vi "Read Measurement Units.vi"(7 "Unit ID (A)":string="A", 8 "error in":errorcluster, 10 "Software Rev":u8, 11 "VISA Session In":refnum<visa-resource-name>="Alicat") -> (0 "error out":errorcluster, 1 "Lock Gas Select":bool, 2 "Measurement Units":T2, 3 "VISA Session Out":refnum<visa-resource-name>)   [LabVIEW 2023]
doc: "Reads the measurement units for the available variables. Measurement units are returned as strings."
panel:
  in  "Gauge (T) or \nDifferential (F)":bool
  out "Measurement Units Intermediate\n(newer revisions)":T1={"Abs. Pressure Units"=1, "Gauge/Diff. Press. Units"=1, "Barometric Press. Units"=1, "Temperature Units"=1, "Volumetric Units"=1, "Mass Units"=1, "Setpoint Units"=1, "Valve Drive Units"=1, "Total Mass Units"=1, "Total Volume Units"=1, "Time Units"=1} {"Setpoint Units" items=["Default"=0, "Unknown"=1, "SuL/m"=2, "SmL/s"=3, "SmL/m"=4, "SmL/h"=5, "SL/s"=6, "SLPM"=7, "SL/h"=8, "SCCS"=11, "SCCM"=12, "Scm3/h"=13, "Sm3/m"=14, "Sm3/h"=15, "Sm3/d"=16, "Sin3/m"=17, "SCFM"=18, "SCFH"=19, "kSCFM"=20, "NuL/m"=32, "NmL/s"=33, "NmL/m"=34, "NmL/h"=35, "NL/s"=36, "NLPM"=37, "NL/h"=38, "NCCS"=41, "NCCM"=42, "Ncm3/h"=43, "Nm3/m"=44, "Nm3/h"=45, "Nm3/d"=46, "count"=62, "%"=63, "mg/s"=64, "mg/m"=65, "g/s"=66, "g/m"=67, "g/h"=68, "kg/m"=69, "kg/h"=70, "oz/s"=71, "oz/m"=72, "lb/m"=73, "lb/h"=74]; "Barometric Press. Units" items=["Default"=0, "Unknown"=1, "Pa"=2, "hPa"=3, "kPa"=4, "MPa"=5, "mbar"=6, "bar"=7, "g/cm2"=8, "kg/cm"=9, "PSI"=10, "PSF"=11, "mTorr"=12, "torr"=13, "mmHg"=14, "inHg"=15, "mmH2O"=16, "mmH2O"=17, "cmH2O"=18, "cmH2O"=19, "inH2O"=20, "inH2O"=21, "atm"=22, "m asl"=23, "ft asl"=24, "V"=61, "count"=62, "%"=63]; "Gauge/Diff. Press. Units" items=["Default"=0, "Unknown"=1, "Pa"=2, "hPa"=3, "kPa"=4, "MPa"=5, "mbar"=6, "bar"=7, "g/cm2"=8, "kg/cm"=9, "PSI"=10, "PSF"=11, "mTorr"=12, "torr"=13, "mmHg"=14, "inHg"=15, "mmH2O"=16, "mmH2O"=17, "cmH2O"=18, "cmH2O"=19, "inH2O"=20, "inH2O"=21, "atm"=22, "m asl"=23, "ft asl"=24, "V"=61, "count"=62, "%"=63]; "Time Units" items=["Default", "Unknown", "h:m:s", "ms", "s", "m", "hour", "day"]; "Total Volume Units" items=["Default"=0, "Unknown"=1, "uL"=2, "mL"=3, "L"=4, "US GAL"=5, "cm3"=6, "m3"=7, "in3"=8, "ft3"=9, "uP"=61]; "Total Mass Units" items=["Default"=0, "Unknown"=1, "SuL"=2, "SmL"=3, "SL"=4, "Scm3"=6, "Sm3"=7, "Sin3"=8, "Sft3"=9, "kSft3"=10, "NuL"=32, "NmL"=33, "NL"=34, "Ncm3"=35, "Nm3"=36, "mg"=64, "g"=65, "kg"=66, "oz"=67, "lb"=68]; "Valve Drive Units" items=["Default"=0, "Unknown"=1, "count"=2, "%"=63]; "Mass Units" items=["Default"=0, "Unknown"=1, "SuL/m"=2, "SmL/s"=3, "SmL/m"=4, "SmL/h"=5, "SL/s"=6, "SLPM"=7, "SL/h"=8, "SCCS"=11, "SCCM"=12, "Scm3/h"=13, "Sm3/m"=14, "Sm3/h"=15, "Sm3/d"=16, "Sin3/m"=17, "SCFM"=18, "SCFH"=19, "kSCFM"=20, "NuL/m"=32, "NmL/s"=33, "NmL/m"=34, "NmL/h"=35, "NL/s"=36, "NLPM"=37, "NL/h"=38, "NCCS"=41, "NCCM"=42, "Ncm3/h"=43, "Nm3/m"=44, "Nm3/h"=45, "Nm3/d"=46, "count"=62, "%"=63, "mg/s"=64, "mg/m"=65, "g/s"=66, "g/m"=67, "g/h"=68, "kg/m"=69, "kg/h"=70, "oz/s"=71, "oz/m"=72, "lb/m"=73, "lb/h"=74]; "Volumetric Units" items=["Default"=0, "Unknown"=1, "uL/m"=2, "mL/s"=3, "mL/m"=4, "mL/h"=5, "L/s"=6, "LPM"=7, "L/h"=8, "US GPM"=9, "US GPH"=10, "CCS"=11, "CCM"=12, "cm3/h"=13, "m3/m"=14, "m3/h"=15, "m3/d"=16, "in3/m"=17, "CFM"=18, "CFH"=19, "count"=62, "%"=63]; "Temperature Units" items=["Default", "Unknown", "°C", "°F", "K", "°Ra"]; "Abs. Pressure Units" items=["Default"=0, "Unknown"=1, "Pa"=2, "hPa"=3, "kPa"=4, "MPa"=5, "mbar"=6, "bar"=7, "g/cm2"=8, "kg/cm"=9, "PSI"=10, "PSF"=11, "mTorr"=12, "torr"=13, "mmHg"=14, "inHg"=15, "mmH2O"=16, "mmH2O"=17, "cmH2O"=18, "cmH2O"=19, "inH2O"=20, "inH2O"=21, "atm"=22, "m asl"=23, "ft asl"=24, "V"=61, "count"=62, "%"=63]}
  out "Measurement Units Intermediate\n(older revisions)":T3={"Pressure Units"=0, "Mass Units"=0, "Temperature Units"=0, "Volume Units"=0, "Totalizer Units"=15, "Totalizer Avg Units"=15} {"Totalizer Units" items=["CC", "uL", "L", "CI", "CF", "CM", "GAL", "mL", "uP", "Lbs", "N/A", "N/A", "N/A", "SCC", "SuL", "SL", "SCI", "SCF", "NCM", "Grams", "Kg", "Lbs", "mg", "SCM", "SmL", "KSCF"]; "Totalizer Avg Units" items=["CCM", "uLPM", "LPM", "CIM", "CFM", "CM/M", "GAL/M", "mLPM", "uP/M", "Lbs/M", "N/A", "N/A", "N/A", "SCCM", "SuLPM", "SLPM", "SCIM", "SCFM", "NCM/M", "Grams/M", "Kg/M", "Lbs/M", "mg/M", "SCM/M", "SmLPM", "KSCFM"]; "Volume Units" items=["CCM"=0, "CCH"=64, "uLPM"=256, "LPS"=320, "LPM"=512, "CM/D"=576, "CIM"=768, "Percent"=832, "CFH"=1024, "Kg/M"=1088, "CM/H"=1280, "Kg/H"=1344, "CFM"=1536, "mLPS"=1600, "GPM"=1792, "CCS"=1856, "GPH"=2048, "mLPH"=2112, "Grams/S"=2304, "Lbs/H"=2368, "Grams/M"=2560, "Grams/H"=2816, "mg/M"=3072, "LPH"=3328, "oz/S"=3584, "mLPM"=3840]; "Temperature Units" items=["C"=0, "K"=16, "F"=32, "R"=48]; "Mass Units" items=["SCCM"=0, "SLPH"=128, "SuLPM"=4096, "SmLPM"=4224, "SLPM"=8192, "Grams/S"=8320, "SCIM"=12288, "SCM/H"=12416, "SCFH"=16384, "SCCH"=16512, "NCM/H"=20480, "NLPH"=20608, "SCFM"=24576, "NLPS"=24704, "Grams/M"=28672, "SCM/D"=28800, "Grams/H"=32768, "NmLPM"=32896, "Kg/M"=36864, "SCCS"=36992, "Kg/H"=40960, "NmLPH"=41088, "Lbs/M"=45056, "SLPS"=45184, "Lbs/H"=49152, "SmLPS"=49280, "mg/M"=53248, "mg/S"=53376, "NLPM"=57344, "NCCM"=61440]; "Pressure Units" items=["PSI", "PSI", "Torr", "Bar", "mBar", "Pascal", "KPa", "MPa", "inHg", "mmHg", "inH2O", "PSID", "mTorr", "cmH2O", "Kg/CM2", "mmH2O"]}
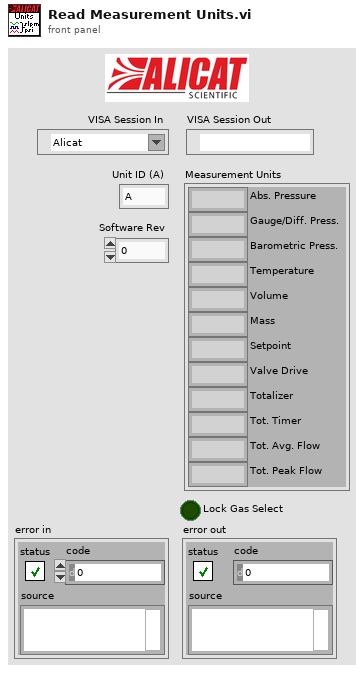
[diagram p1: front panel]
types:
  T1 = cluster{"Abs. Pressure Units":u16, "Gauge/Diff. Press. Units":u16, "Barometric Press. Units":u16, "Temperature Units":u16, "Volumetric Units":u16, "Mass Units":u16, "Setpoint Units":u16, "Valve Drive Units":u16, "Total Mass Units":u16, "Total Volume Units":u16, "Time Units":u16}
  T2 = cluster{"Abs. Pressure":string, "Gauge/Diff. Press.":string, "Barometric Press.":string, "Temperature":string, "Volume":string, "Mass":string, "Setpoint":string, "Valve Drive":string, "Totalizer":string, "Tot. Timer":string, "Tot. Avg. Flow":string, "Tot. Peak Flow":string}
  T3 = cluster{"Pressure Units":i32, "Mass Units":i32, "Temperature Units":i32, "Volume Units":i32, "Totalizer Units":u16, "Totalizer Avg Units":u16}
  T4 = cluster{"Pressure":i32, "Mass":i32, "Temperature":i32, "Volume":i32, "Totalizer Units":u16, "Totalizer Avg Units":u16}
  T5 = typedef "LVStringsAndValuesArrayTypeDef_U16.ctl" = cluster{"String":string, "Value":u16}[]
  T6 = cluster{"Controller Select":u16, "SetPoint Source":enum8{"Serial", "Local", "Analog", "Unknown"}, "AutoTare":enum16{"Disabled", "Enabled"}}
  T7 = typedef "LVStringsAndValuesArrayTypeDef_I32.ctl" = cluster{"String":string, "Value":i32}[]
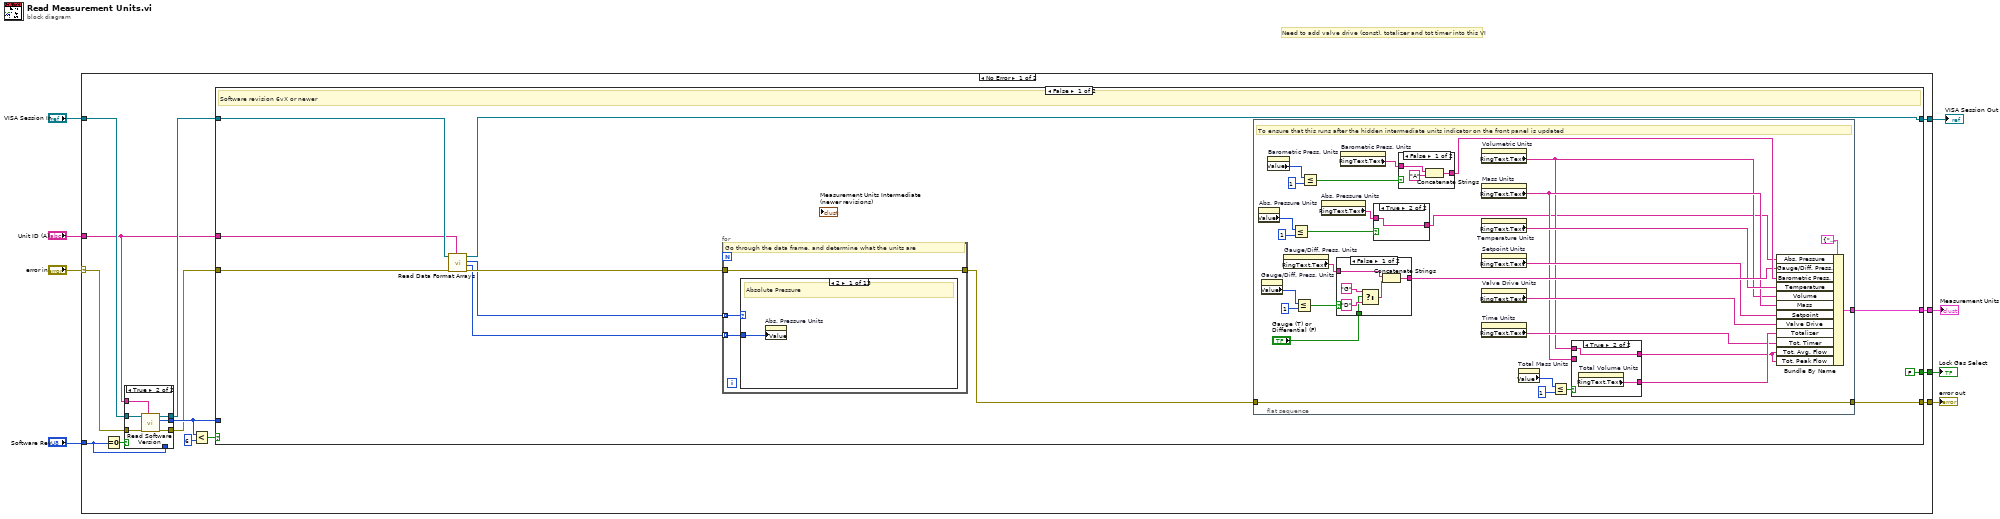
[diagram p0: block diagram]
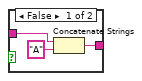
[diagram p5: hidden frame]
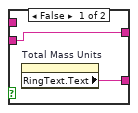
[diagram p6: hidden frame]
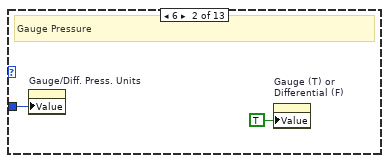
[diagram p7: hidden frame]
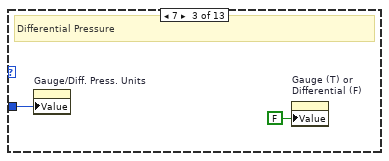
[diagram p8: hidden frame]
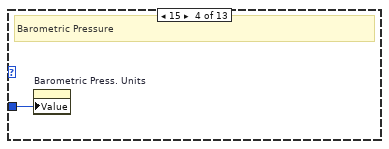
[diagram p9: hidden frame]
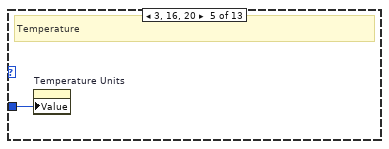
[diagram p10: hidden frame]
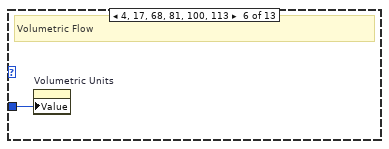
[diagram p11: hidden frame]
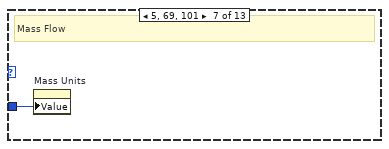
[diagram p12: hidden frame]
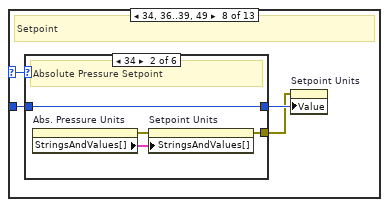
[diagram p13: hidden frame]
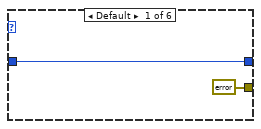
[diagram p14: hidden frame]
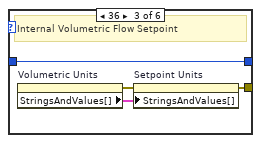
[diagram p15: hidden frame]
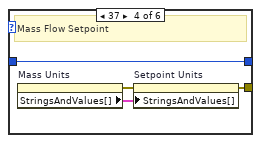
[diagram p16: hidden frame]
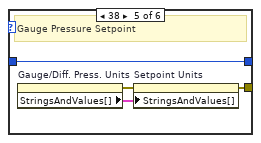
[diagram p17: hidden frame]
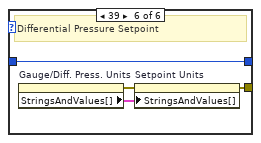
[diagram p18: hidden frame]
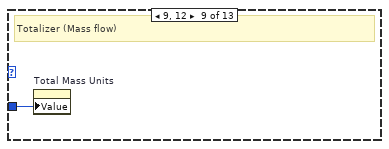
[diagram p19: hidden frame]
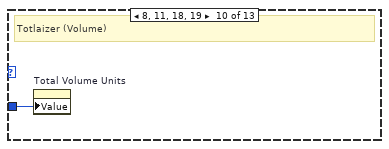
[diagram p20: hidden frame]
diagram:
  # "Need to add valve drive (const), totalizer and tot timer into this VI"
  n1 = case shown="No Error" "error in" {
    selector: "error in" -> [w11 w253]
    tunnel: [w22 TRUE ("Lock Gas Select")] -> w8
    tunnel: [w21 w253] -> w7
    tunnel: "Software Rev" -> [w15 _]
    tunnel: "Unit ID (A)" -> [w9 _]
    tunnel: "VISA Session In" -> [w10 w256]
    tunnel: [w19 w256] -> w3
    tunnel: [w18 T2 {"Abs. Pressure"="", "Gauge/Diff. Press."="", "Barometric Press."="", "Temperature"="", "Volume"="", "Mass"="", "Setpoint"="", "Valve Drive"="", "Totalizer"="", "Tot. Timer"="", "Tot. Avg. Flow"="", "Tot. Peak Flow"=""} ("Measurement Units")] -> w2
    frame No Error {
      n2 = Equal To 0?(x=w15) -> (x = 0?=w16:bool)
      n3 = case shown="True" w16 {
        tunnel: w11 -> [w24 w31]
        tunnel: w10 -> [w23 w30]
        tunnel: w9 -> [_ w29]
        tunnel: [w24 w28] -> w12
        tunnel: [w23 w27] -> w13
        tunnel: [w25 w26] -> w14
        tunnel: w15 -> [w25 _]
        frame False {
        }
        frame True {
          n4 = call "Read Software Version.vi"("Unit ID (A)"=w29, "error in"=w31, "VISA Session In"=w30) -> ("error out"=w28:errorcluster, "Software Version"=w26:u8, "VISA Session Out"=w27:refnum<visa-resource-name>)  [unwired: 6 in]
        }
      }
      n5 = Less?(x=w14, y=u8 6) -> (x < y?=w20:bool)
      n6 = case shown="False" w20 {
        tunnel: [FALSE ("Lock Gas Select") w157] -> w22
        tunnel: w12 -> [w38 w148]
        tunnel: [w40 w143] -> w21
        tunnel: w14 -> [_ w152]
        tunnel: w13 -> [w37 w149]
        tunnel: w9 -> [w36 w138]
        tunnel: [w35 w145] -> w19
        tunnel: [w39 w144] -> w18
        frame False {
          # "Software revision 6vX or newer"
          n7 = call "Read Data Format Arrays.vi"("Unit ID (A)"=w36, "error in (no error)"=w38, "VISA Session In"=w37) -> ("error out"=w34:errorcluster, "Units Array"=w32:u16[], "Data Type Array"=w33:u16[], "VISA Session Out"=w35:refnum<visa-resource-name>)  [unwired: 5 in]
          n8 = for {
            tunnel: w32 -> [w93] mode=indexing
            tunnel: w33 -> [w94] mode=indexing
            tunnel: [w92] -> w41
            tunnel: w34 -> [w92]
            # "Go through the data frame, and determine what the units are"
            n9 = case shown="2" w94 {
              selector: w94 -> [_ _ _ _ _ _ _ w105 _ _ _ _ _]
              tunnel: w93 -> [w95 w97 w99 w100 w101 w102 w103 w104 w130 w131 w132 w133 _]
              frame 2 {
                # "Absolute Pressure"
                n10 = property on="Abs. Pressure Units" class="Ring (strict)"("Value"=w95) -> ()  [unwired: 2 in, 2 out]
              }
              frame 6 {
                # "Gauge Pressure"
                n11 = property on="Gauge/Diff. Press. Units" class="Ring (strict)"("Value"=w97) -> ()  [unwired: 2 in, 2 out]
                n12 = property on="Gauge (T) or \nDifferential (F)" class="Bool (strict)"("Value"=TRUE ("Gauge")) -> ()  [unwired: 2 in, 2 out]
              }
              frame 7 {
                # "Differential Pressure"
                n13 = property on="Gauge/Diff. Press. Units" class="Ring (strict)"("Value"=w99) -> ()  [unwired: 2 in, 2 out]
                n14 = property on="Gauge (T) or \nDifferential (F)" class="Bool (strict)"("Value"=FALSE ("Gauge")) -> ()  [unwired: 2 in, 2 out]
              }
              frame 15 {
                # "Barometric Pressure"
                n15 = property on="Barometric Press. Units" class="Ring (strict)"("Value"=w100) -> ()  [unwired: 2 in, 2 out]
              }
              frame 3, 16, 20 {
                # "Temperature"
                n16 = property on="Temperature Units" class="Ring (strict)"("Value"=w101) -> ()  [unwired: 2 in, 2 out]
              }
              frame 4, 17, 68, 81, 100, 113 {
                # "Volumetric Flow"
                n17 = property on="Volumetric Units" class="Ring (strict)"("Value"=w102) -> ()  [unwired: 2 in, 2 out]
              }
              frame 5, 69, 101 {
                # "Mass Flow"
                n18 = property on="Mass Units" class="Ring (strict)"("Value"=w103) -> ()  [unwired: 2 in, 2 out]
              }
              frame 34, 36..39, 49 {
                # "Setpoint"
                n19 = case shown="34" w105 {
                  tunnel: [w108 w110 w114 w118 w122 w126] -> w107
                  tunnel: [errorcluster {"status"=FALSE, "code"=0, "source"=""} ("error out") w111 w115 w119 w123 w127] -> w106
                  tunnel: w104 -> [w108 w110 w114 w118 w122 w126]
                  frame Default {
                  }
                  frame 34 {
                    # "Absolute Pressure Setpoint"
                    n20 = property on="Abs. Pressure Units" class="Ring (strict)"() -> (error out=w113:errorcluster, "StringsAndValues[]"=w112:T5)  [unwired: 2 in, 1 out]
                    n21 = property on="Setpoint Units" class="Ring (strict)"(error in=w113, "StringsAndValues[]"=w112) -> (error out=w111:errorcluster)  [unwired: 1 in, 1 out]
                  }
                  frame 36 {
                    # "Internal Volumetric Flow Setpoint"
                    n22 = property on="Volumetric Units" class="Ring (strict)"() -> (error out=w117:errorcluster, "StringsAndValues[]"=w116:T5)  [unwired: 2 in, 1 out]
                    n23 = property on="Setpoint Units" class="Ring (strict)"(error in=w117, "StringsAndValues[]"=w116) -> (error out=w115:errorcluster)  [unwired: 1 in, 1 out]
                  }
                  frame 37 {
                    # "Mass Flow Setpoint"
                    n24 = property on="Mass Units" class="Ring (strict)"() -> (error out=w121:errorcluster, "StringsAndValues[]"=w120:T5)  [unwired: 2 in, 1 out]
                    n25 = property on="Setpoint Units" class="Ring (strict)"(error in=w121, "StringsAndValues[]"=w120) -> (error out=w119:errorcluster)  [unwired: 1 in, 1 out]
                  }
                  frame 38 {
                    # "Gauge Pressure Setpoint"
                    n26 = property on="Gauge/Diff. Press. Units" class="Ring (strict)"() -> (error out=w125:errorcluster, "StringsAndValues[]"=w124:T5)  [unwired: 2 in, 1 out]
                    n27 = property on="Setpoint Units" class="Ring (strict)"(error in=w125, "StringsAndValues[]"=w124) -> (error out=w123:errorcluster)  [unwired: 1 in, 1 out]
                  }
                  frame 39 {
                    # "Differential Pressure Setpoint"
                    n28 = property on="Gauge/Diff. Press. Units" class="Ring (strict)"() -> (error out=w129:errorcluster, "StringsAndValues[]"=w128:T5)  [unwired: 2 in, 1 out]
                    n29 = property on="Setpoint Units" class="Ring (strict)"(error in=w129, "StringsAndValues[]"=w128) -> (error out=w127:errorcluster)  [unwired: 1 in, 1 out]
                  }
                }
                n30 = property on="Setpoint Units" class="Ring (strict)"(error in=w106, "Value"=w107) -> ()  [unwired: 1 in, 2 out]
              }
              frame 9, 12 {
                # "Totalizer (Mass flow)"
                n31 = property on="Total Mass Units" class="Ring (strict)"("Value"=w130) -> ()  [unwired: 2 in, 2 out]
              }
              frame 8, 11, 18, 19 {
                # "Totlaizer (Volume)"
                n32 = property on="Total Volume Units" class="Ring (strict)"("Value"=w131) -> ()  [unwired: 2 in, 2 out]
              }
              frame 13 {
                # "Valve Drive"
                n33 = property on="Valve Drive Units" class="Ring (strict)"("Value"=w132) -> ()  [unwired: 2 in, 2 out]
              }
              frame 10, 14 {
                # "Time"
                n34 = property on="Time Units" class="Ring (strict)"("Value"=w133) -> ()  [unwired: 2 in, 2 out]
              }
              frame Default {
              }
            }
          }
          n35 = flat-sequence {
            tunnel: w41 -> [w59]
            tunnel: [w59] -> w40
            tunnel: [w44] -> w39
            frame #0 {
              # "To ensure that this runs after the hidden intermediate units indicator on the front panel is updated"
              n36 = property on="Abs. Pressure Units" class="Ring (strict)"() -> ("Value"=w65:u16)  [unwired: 2 in, 2 out]
              n37 = property on="Gauge/Diff. Press. Units" class="Ring (strict)"() -> ("Value"=w66:u16)  [unwired: 2 in, 2 out]
              n38 = property on="Barometric Press. Units" class="Ring (strict)"() -> ("Value"=w69:u16)  [unwired: 2 in, 2 out]
              n39 = property on="Gauge/Diff. Press. Units" class="Ring (strict)"() -> ("RingText.Text"=w56:string)  [unwired: 2 in, 2 out]
              n40 = Less Or Equal?(x=w65, y=u16 1) -> (x <= y?=w63:bool)
              n41 = Less Or Equal?(x=w66, y=u16 1) -> (x <= y?=w57:bool)
              n42 = Less Or Equal?(x=w69, y=u16 1) -> (x <= y?=w60:bool)
              n43 = property on="Abs. Pressure Units" class="Ring (strict)"() -> ("RingText.Text"=w62:string)  [unwired: 2 in, 2 out]
              n44 = case shown="False" w57 {
                tunnel: w56 -> [w78 w79]
                tunnel: [w77 w79] -> w54
                tunnel: "Gauge (T) or \nDifferential (F)" -> [w73 _]
                frame False {
                  n45 = Select(t="G" ("string"), s=w73, f="D" ("string")) -> (s? t:f=w74:string)
                  n46 = Concatenate Strings(w78, w74) -> (w77:string)
                }
                frame True {
                }
              }
              n47 = property on="Barometric Press. Units" class="Ring (strict)"() -> ("RingText.Text"=w61:string)  [unwired: 2 in, 2 out]
              n48 = case shown="True" w63 {
                tunnel: w62 -> [w85 w87]
                tunnel: [w84 w87] -> w43
                frame False {
                  n49 = Concatenate Strings(w85, "A" ("string")) -> (w84:string)
                }
                frame True {
                }
              }
              n50 = case shown="False" w60 {
                tunnel: w61 -> [w81 w83]
                tunnel: [w80 w83] -> w55
                frame False {
                  n51 = Concatenate Strings(w81, "A" ("string")) -> (w80:string)
                }
                frame True {
                }
              }
              n52 = property on="Volumetric Units" class="Ring (strict)"() -> ("RingText.Text"=w46:string)  [unwired: 2 in, 2 out]
              n53 = property on="Mass Units" class="Ring (strict)"() -> ("RingText.Text"=w47:string)  [unwired: 2 in, 2 out]
              n54 = property on="Temperature Units" class="Ring (strict)"() -> ("RingText.Text"=w53:string)  [unwired: 2 in, 2 out]
              n55 = property on="Setpoint Units" class="Ring (strict)"() -> ("RingText.Text"=w50:string)  [unwired: 2 in, 2 out]
              n56 = property on="Valve Drive Units" class="Ring (strict)"() -> ("RingText.Text"=w49:string)  [unwired: 2 in, 2 out]
              n57 = property on="Time Units" class="Ring (strict)"() -> ("RingText.Text"=w48:string)  [unwired: 2 in, 2 out]
              n58 = property on="Total Mass Units" class="Ring (strict)"() -> ("Value"=w70:u16)  [unwired: 2 in, 2 out]
              n59 = Less Or Equal?(x=w70, y=u16 1) -> (x <= y?=w71:bool)
              n60 = case shown="True" w71 {
                tunnel: [w89 w91] -> w51
                tunnel: w47 -> [w88 _]
                tunnel: w46 -> [_ w90]
                tunnel: [w88 w90] -> w45
                frame False {
                  n61 = property on="Total Mass Units" class="Ring (strict)"() -> ("RingText.Text"=w89:string)  [unwired: 2 in, 2 out]
                }
                frame True {
                  n62 = property on="Total Volume Units" class="Ring (strict)"() -> ("RingText.Text"=w91:string)  [unwired: 2 in, 2 out]
                }
              }
              n63 = Bundle By Name(cluster=T2 {"Abs. Pressure"="", "Gauge/Diff. Press."="", "Barometric Press."="", "Temperature"="", "Volume"="", "Mass"="", "Setpoint"="", "Valve Drive"="", "Totalizer"="", "Tot. Timer"="", "Tot. Avg. Flow"="", "Tot. Peak Flow"=""} ("Measurement Units"), "Abs. Pressure"=w43, "Gauge/Diff. Press."=w54, "Barometric Press."=w55, "Temperature"=w53, "Volume"=w46, "Mass"=w47, "Setpoint"=w50, "Valve Drive"=w49, "Totalizer"=w51, "Tot. Timer"=w48, "Tot. Avg. Flow"=w45, "Tot. Peak Flow"=w45) -> (w44:T2)
            }
          }
        }
        frame True {
          # "If true mass units on an \nold board: lock gas select"
          # "Software revision 5vX or older"
          n64 = call "Read Register.vi"("Unit ID (A)"=w138, "error in"=w148, "Register address"=u16 45, "VISA Session In"=w149) -> ("error out"=w142:errorcluster, "Register Value (I32)"=w147:i32, "VISA Session Out"=w140:refnum<visa-resource-name>)  [unwired: 5 in]
          n65 = call "Read Output Definitions and Controller Options.vi"("Unit ID (A)"=w138, "error in"=w142, "VISA Session In"=w140) -> ("error out"=w141:errorcluster, "Read/Write Options"=w137:T6, "VISA Session Out"=w139:refnum<visa-resource-name>)  [unwired: 5 in, 1 out]
          n66 = Unbundle By Name(w137) -> ("Controller Select"=w136:u16)
          n67 = call "Read Totalizer Units and Decimals.vi"("Unit ID (A)"=w138, "error in"=w141, "VISA Session In"=w139) -> ("error out"=w146:errorcluster, "Totalizer Units"=w135:string, "VISA Session Out"=w145:refnum<visa-resource-name>)  [unwired: 4 in, 2 out]
          n68 = property on="Mass Units" class="Ring (strict)"(error in=w146) -> (error out=w156:errorcluster, "StringsAndValues[]"=w194:T7)  [unwired: 1 in, 1 out]
          n69 = for {
            tunnel: w194 -> [w252] mode=indexing
            tunnel: [w251] -> w170 mode=indexing
            n70 = Unbundle By Name(w252) -> ("Value"=w251:i32)
          }
          n71 = property on="Volume Units" class="Ring (strict)"(error in=w156) -> (error out=w155:errorcluster, "StringsAndValues[]"=w185:T7)  [unwired: 1 in, 1 out]
          n72 = Less Or Equal?(x=w170, y=w147) -> (x <= y?=w193:bool[])
          n73 = Boolean To (0,1)(Boolean=w193) -> (0, 1=w192:i16[])
          n74 = To Long Integer(number=w192) -> (32bit integer=w191:i32[])
          n75 = Multiply(x=w170, y=w191) -> (x*y=w190:i32[])
          n76 = for {
            tunnel: w185 -> [w250] mode=indexing
            tunnel: [w249] -> w168 mode=indexing
            n77 = Unbundle By Name(w250) -> ("Value"=w249:i32)
          }
          n78 = Array Max & Min(array=w190) -> (max value=w164:i32, max index (indices)=w169:i32)  [unwired: 2 out]
          n79 = Subtract(x=w147, y=w164) -> (x-y=w184:i32)
          n80 = property on="Temperature Units" class="Ring (strict)"(error in=w155) -> (error out=w154:errorcluster, "StringsAndValues[]"=w183:T7)  [unwired: 1 in, 1 out]
          n81 = Less Or Equal?(x=w168, y=w184) -> (x <= y?=w186:bool[])
          n82 = Boolean To (0,1)(Boolean=w186) -> (0, 1=w187:i16[])
          n83 = To Long Integer(number=w187) -> (32bit integer=w188:i32[])
          n84 = Multiply(x=w168, y=w188) -> (x*y=w189:i32[])
          n85 = for {
            tunnel: w183 -> [w248] mode=indexing
            tunnel: [w247] -> w167 mode=indexing
            n86 = Unbundle By Name(w248) -> ("Value"=w247:i32)
          }
          n87 = Array Max & Min(array=w189) -> (max value=w163:i32)  [unwired: 3 out]
          n88 = Subtract(x=w184, y=w163) -> (x-y=w173:i32)
          n89 = property on="Pressure Units" class="Ring (strict)"(error in=w154) -> (error out=w153:errorcluster, "StringsAndValues[]"=w174:T7)  [unwired: 1 in, 1 out]
          n90 = Less Or Equal?(x=w167, y=w173) -> (x <= y?=w182:bool[])
          n91 = Boolean To (0,1)(Boolean=w182) -> (0, 1=w181:i16[])
          n92 = To Long Integer(number=w181) -> (32bit integer=w180:i32[])
          n93 = Multiply(x=w167, y=w180) -> (x*y=w179:i32[])
          n94 = for {
            tunnel: w174 -> [w246] mode=indexing
            tunnel: [w245] -> w166 mode=indexing
            n95 = Unbundle By Name(w246) -> ("Value"=w245:i32)
          }
          n96 = Array Max & Min(array=w179) -> (max value=w162:i32)  [unwired: 3 out]
          n97 = Subtract(x=w173, y=w162) -> (x-y=w172:i32)
          n98 = Less Or Equal?(x=w166, y=w172) -> (x <= y?=w175:bool[])
          n99 = Boolean To (0,1)(Boolean=w175) -> (0, 1=w176:i16[])
          n100 = To Long Integer(number=w176) -> (32bit integer=w177:i32[])
          n101 = Multiply(x=w166, y=w177) -> (x*y=w178:i32[])
          n102 = Array Max & Min(array=w178) -> (max value=w161:i32)  [unwired: 3 out]
          n103 = Subtract(x=w172, y=w161) -> (x-y=w171:i32)
          n104 = Not Equal To 0?(x=w171) -> (x != 0?=w165:bool)
          n105 = case shown="True" w165 {
            tunnel: w170 -> [_ w244]
            tunnel: w169 -> [_ w242]
            tunnel: w168 -> [_ w237]
            tunnel: w167 -> [_ w231]
            tunnel: w166 -> [_ w225]
            tunnel: w164 -> [w218 _]
            tunnel: w163 -> [w217 _]
            tunnel: w162 -> [w216 _]
            tunnel: w161 -> [w215 _]
            tunnel: [w218 w220] -> w195
            tunnel: [w217 w224] -> w158
            tunnel: [w216 w223] -> w160
            tunnel: [w215 w222] -> w159
            tunnel: w147 -> [_ w219]
            frame False {
            }
            frame True {
              # "If remainder =/= 0, then the value used a combination of bits and needs to be re-checked"
              n106 = Decrement(x=w242) -> (x-1=w243:i32)
              n107 = Index Array(array=w244, index=w243) -> (element=w220:i32)
              n108 = Subtract(x=w219, y=w220) -> (x-y=w221:i32)
              n109 = Less Or Equal?(x=w237, y=w221) -> (x <= y?=w241:bool[])
              n110 = Boolean To (0,1)(Boolean=w241) -> (0, 1=w240:i16[])
              n111 = To Long Integer(number=w240) -> (32bit integer=w239:i32[])
              n112 = Multiply(x=w237, y=w239) -> (x*y=w238:i32[])
              n113 = Array Max & Min(array=w238) -> (max value=w224:i32)  [unwired: 3 out]
              n114 = Subtract(x=w221, y=w224) -> (x-y=w232:i32)
              n115 = Less Or Equal?(x=w231, y=w232) -> (x <= y?=w233:bool[])
              n116 = Boolean To (0,1)(Boolean=w233) -> (0, 1=w234:i16[])
              n117 = To Long Integer(number=w234) -> (32bit integer=w235:i32[])
              n118 = Multiply(x=w231, y=w235) -> (x*y=w236:i32[])
              n119 = Array Max & Min(array=w236) -> (max value=w223:i32)  [unwired: 3 out]
              n120 = Subtract(x=w232, y=w223) -> (x-y=w226:i32)
              n121 = Less Or Equal?(x=w225, y=w226) -> (x <= y?=w230:bool[])
              n122 = Boolean To (0,1)(Boolean=w230) -> (0, 1=w229:i16[])
              n123 = To Long Integer(number=w229) -> (32bit integer=w228:i32[])
              n124 = Multiply(x=w225, y=w228) -> (x*y=w227:i32[])
              n125 = Array Max & Min(array=w227) -> (max value=w222:i32)  [unwired: 3 out]
            }
          }
          n126 = Bundle By Name(cluster=T4 {"Pressure"=0, "Mass"=0, "Temperature"=0, "Volume"=0, "Totalizer Units"=15, "Totalizer Avg Units"=15} ("Measurement Units Intermediate\n(older revisions)"), "Mass"=w195, "Volume"=w158, "Temperature"=w160, "Pressure"=w159) -> (w151:T4)
          n127 = call "Gas Select Lock Check.vi"("error in"=w153, "Software Rev"=w152, "Volumetric Units Code"=w158, "Mass Units Code"=w195) -> ("error out"=w143:errorcluster, "Lock Gas Select"=w157:bool)  [unwired: 6 in]
          n128 = flat-sequence {
            tunnel: w151 -> [w207]
            tunnel: [w206] -> w144
            tunnel: w136 -> [w204]
            tunnel: w135 -> [w196]
            frame #0 {
              # "Flat sequence to force this code to execute after the units are determined"
              n129 = property on="Pressure Units" class="Ring (strict)"() -> ("RingText.Text"=w203:string)  [unwired: 2 in, 2 out]
              n130 = property on="Temperature Units" class="Ring (strict)"() -> ("RingText.Text"=w208:string)  [unwired: 2 in, 2 out]
              n131 = property on="Volume Units" class="Ring (strict)"() -> ("RingText.Text"=w202:string)  [unwired: 2 in, 2 out]
              n132 = property on="Mass Units" class="Ring (strict)"() -> ("RingText.Text"=w201:string)  [unwired: 2 in, 2 out]
              n133 = Concatenate Strings(w196, "/M" ("string")) -> (w197:string)
              n134 = case shown="0, Default" w204 {
                tunnel: w203 -> [_ w212 _ _]
                tunnel: w202 -> [_ _ w213 _]
                tunnel: w201 -> [_ _ _ w214]
                tunnel: ["Unknown" ("RingText.Text") w212 w213 w214] -> w200
                frame 0, Default {
                }
                frame 34, 38, 39 {
                }
                frame 36 {
                }
                frame 37 {
                }
              }
              n135 = Bundle By Name(cluster=T2 {"Abs. Pressure"="", "Gauge/Diff. Press."="", "Barometric Press."="", "Temperature"="", "Volume"="", "Mass"="", "Setpoint"="", "Valve Drive"="", "Totalizer"="", "Tot. Timer"="", "Tot. Avg. Flow"="", "Tot. Peak Flow"=""} ("Measurement Units"), "Setpoint"=w200, "Abs. Pressure"=w203, "Gauge/Diff. Press."=w203, "Barometric Press."="N/A", "Temperature"=w208, "Volume"=w202, "Mass"=w201, "Valve Drive"="%", "Totalizer"=w196, "Tot. Avg. Flow"=w197, "Tot. Peak Flow"=w196, "Tot. Timer"="h:m:s") -> (w206:T2)
              "Measurement Units Intermediate\n(older revisions)" <- w207
            }
          }
        }
      }
    }
    frame Error {
    }
  }
  "error out" <- w7
  "VISA Session Out" <- w3
  "Lock Gas Select" <- w8
  "Measurement Units" <- w2
